vi "cvt tag to tag bus tag.vi"(11 "CVT Tags":T1[](array[typedef])) -> (3 "TB Tags":refnum<class "tag descriptor.lvclass">[](array[class]))   [LabVIEW 2013, in "CVT Engine Configuration.lvclass"]
uses:
  CVT Engine Configuration.lvclass
  <vilib>/NI/Current Value Table/Type Defs/Single Tag.ctl
  <vilib>/NI/Current Value Table/Type Defs/Data Types.ctl
  <vilib>/NI/Tag Bus/tag/tag descriptor.lvclass
  <vilib>/NI/Current Value Table/Current Value Table.lvlib
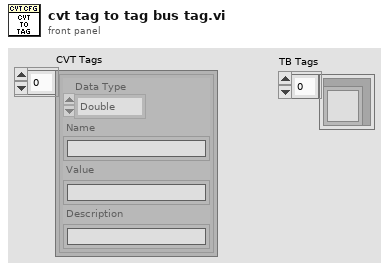
[diagram p1: front panel]
types:
  T1 = typedef "Current Value Table.lvlib/Single Tag.ctl" = cluster{"Data Type":T2, "Name":string, "Value":string, "Description":string}
  T2 = typedef "Current Value Table.lvlib/Data Types.ctl" = enum16{"Double", "Single", "I64", "I32", "I16", "I8", "U64", "U32", "U16", "U8", "String", "Boolean", "Array of U8", "Array of U16", "Array of U32", "Array of U64", "Array of I64", "Array of I32", "Array of I16", "Array of I8", "Array of Double", "Array of Single", "Array of Boolean", "Array of String"}
  T3 = typedef "tag bus.lvlib/tag descriptor.lvclass/Data Type.ctl" = enum16{"Double", "Single", "I64", "I32", "I16", "I8", "U64", "U32", "U16", "U8", "Boolean", "String", "Array of Double", "Array of Single", "Array of I64", "Array of I32", "Array of I16", "Array of I8", "Array of U64", "Array of U32", "Array of U16", "Array of U8", "Array of Boolean", "Array of String"}
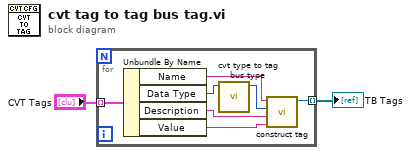
[diagram p0: block diagram]
diagram:
  n1 = for {
    tunnel: "CVT Tags" -> [w9] mode=indexing
    tunnel: [w8] -> w1 mode=indexing
    n2 = Unbundle By Name(w9) -> ("Name"=w7:string, "Data Type"=w4:T2, "Description"=w6:string, "Value"=w5:string)
    n3 = call "cvt type to tag bus type.vi"("cvt type"=w4) -> ("Data Type"=w3:T3)  [unwired: 10 in]
    n4 = call <vilib>:"construct tag.vi"("raw default"=w5, "metadata"=w6, "data type"=w3, "name"=w7) -> ("system tag out"=w8:refnum<class "tag descriptor.lvclass">)  [unwired: 6 in, 1 out]
  }
  "TB Tags" <- w1
